vi "Compressor With Cylinder.vi"() -> ()   [LabVIEW 2013]
doc: "Compressor with Cylinder \n\nThis example shows how to control a compressor, extend and retract a cylinder, and optionally use a limit switch to retract automatically.\n\nThis example works with the NI 9403 module connected to a Digital Sidecar. The Digital Sidecar should have 12V applied to the WAGO connector. A SPIKE relay is used to turn the compressor on and off. The PWM type input on the SPIKE should be wired to RELAY 1 on the Digital Sidecar. The GND and 12V inputs on the SPIKE should get power from the battery through a 20A fuse on the Power Distribution Board. The M+ and M- outputs from the SPIKE should be wired to the compressor. Wire M+ to the red compressor wire, and M- to the black compressor wire. The Pressure Switch is wired to DIGITAL I/O 1. This input determines when the SPIKE relay gets energized to run the compressor. The Limit Switch is wired to DIGITAL I/O 2. It causes the cylinder to retract when the Auto Retract button is pressed.\n\nThis example also uses the Solenoid Breakout connected to the NI 9472 to control the SMC double solenoid valve. From the Solenoid Breakout, channel 1 is wired to terminal A on the valve, and channel 2 is wired to terminal B on the valve.\n\nRefer to the Pneumatics Manual for air connections. Your pneumatics setup should include a compressor, pressure switch, tank, regulator, valve, flow controls, cylinder, plug valve, etc.\n\nTo run this example you should have a pneumatic system with air pressure connected to the P input on the SMC double solenoid valve. The A output of the valve should be connected via a flow control to the backend of a cylinder. The B output of the valve should be connected via a flow control to the frontend of a cylinder. When the cylinder is extended, it should physically depress the Limit Switch.\n\nWith the VI running, pressing the Extend button will push the cylinder shaft out, and pressing the Retract button will pull it back. Notice that the Extend and Retract buttons have their Mechanical Action set to Latch When Pressed. This means they stay pressed (ON) until they are read by the program, then they return to the OFF position. This works because once the SMC solenoid valve is pulled one direction, it stays in that position until it is pulled in the opposite direction - it only needs to be momentarily energized. The Auto Retract button can be used to make the cylinder return automatically. With the Auto Retract button ON, pressing the Extend button will push the cylinder out, and it will retract when it hits the limit switch."
uses:
  <vilib>/Rock Robotics/WPI/Solenoid/WPI_SolenoidChannel.ctl
  <vilib>/Rock Robotics/SystemInterfaces/DIO/FPGA_DIOChannel.ctl
  <vilib>/Rock Robotics/SystemInterfaces/DIO/FPGA_DIORelayChannel.ctl
  <vilib>/Rock Robotics/SystemInterfaces/Typedef/FPGA_TypedefDigitalModule.ctl
  <vilib>/Rock Robotics/SystemInterfaces/Typedef/FPGA_TypedefSolenoidModule.ctl
  <vilib>/Rock Robotics/WPI/Solenoid/WPI_SolenoidValue.ctl
  <vilib>/Rock Robotics/WPI/Solenoid/WPI_SolenoidOpenDouble.vi
  <vilib>/Rock Robotics/WPI/Solenoid/WPI_SolenoidSetEnum.vi
panel:
  in  "Boolean":bool
  in  "Limit_Switch":T1=enum."DIO 10"
  in  "2nd_position":bool
  in  "Shooter":bool
  in  "Load":bool
  in  "Small_Cylinder_Extend":T2=enum."Solenoid 4"
  in  "Small_Cylinder_Retract":T2=enum."Solenoid 3"
  out "Compressor Running?":bool
  in  "Solenoid Module":T3
  in  "Large_Cylinder_Extend":T2=enum."Solenoid 2"
  in  "Switch and Relay Module":T4
  in  "RelayChannel":T5=enum."Relay 2"
  in  "Pressure Switch Channel":T1=enum."DIO 5"
  in  "Large_Cylinder_Retract":T2
  out "Compressor Enabled?":bool
  in  "stop":bool
  # "Set these inputs before running."
  # "These can be set while running."
  # "Output information."
  # "Wiring Diagram for Digital Sidecar connected to an NI 9403"
  # "when extended, the cylinder should depress this"
  # "Limit\nSwitch"
  # "(-)"
  # "B"
  # "A"
  # "8\n7\n6\n5\n4\n3\n2\n1"
  # "RELAY"
  # "Pressure\nSwitch"
  # "Connect\nPower\nHere"
  # "GND"
  # "M-"
  # "Connect\nCompressor\nHere"
  # "SPIKE"
  # "12V"
  # "M+"
  # "B"
  # "20A"
  # "fuse"
  # "SPIKE Relay"
  # "PWM cable"
  # "COM"
  # "NC"
  # "NO"
  # "NC"
  # "C"
  # "PWR"
  # "SIG"
  # "(-)"
  # "14\n13\n12\n11\n10\n9\n8\n7\n6\n5\n4\n3\n2\n1"
  # "DIGITAL I/O"
  # "Digital Sidecar"
  # "Wiring Diagram for Solenoid Breakout connected to an NI 9472"
  # "GND"
  # "SIG"
  # "8\n7\n6\n5\n4\n3\n2\n1"
  # "+"
  # "12V from\nbattery"
  # "-"
  # "tubing port for retract side of cylinder"
  # "tubing port for extend side of cylinder"
  # "\"power good\"\n  LED"
  # "SMC double solenoid valve"
  # "B"
  # "A"
  # "B"
  # "A"
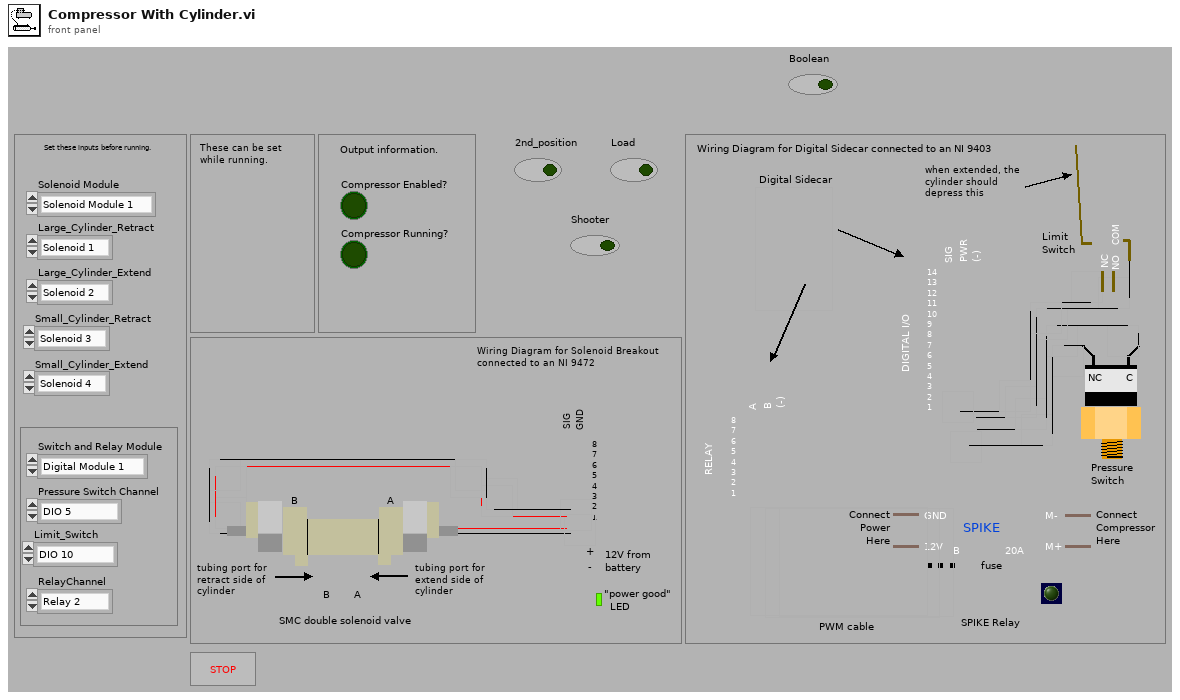
[diagram p1: front panel]
types:
  T1 = typedef "FPGA_DIOChannel.ctl" = enum8{"DIO 1", "DIO 2", "DIO 3", "DIO 4", "DIO 5", "DIO 6", "DIO 7", "DIO 8", "DIO 9", "DIO 10", "DIO 11", "DIO 12", "DIO 13", "DIO 14", "Invalid"}
  T2 = typedef "WPI_SolenoidChannel.ctl" = enum8{"Solenoid 1", "Solenoid 2", "Solenoid 3", "Solenoid 4", "Solenoid 5", "Solenoid 6", "Solenoid 7", "Solenoid 8", "Invalid"}
  T3 = typedef "FPGA_TypedefSolenoidModule.ctl" = enum16{"Solenoid Module 1", "Solenoid Module 2"}
  T4 = typedef "FPGA_TypedefDigitalModule.ctl" = enum16{"Digital Module 1", "Digital Module 2"}
  T5 = typedef "FPGA_DIORelayChannel.ctl" = enum8{"Relay 1", "Relay 2", "Relay 3", "Relay 4", "Relay 5", "Relay 6", "Relay 7", "Relay 8", "Invalid"}
  T6 = typedef "WPI_CompressorDevRef.ctl" = cluster{"DevStatus":errorcluster, "DigitalInputDevRef":T7, "RelayDevRef":T8}
  T7 = typedef "WPI_DigitalInputDevRef.ctl" = cluster{"DevStatus":errorcluster, "DIO Channel":T1, "Digital Module":T4}
  T8 = typedef "WPI_RelayDevRef.ctl" = cluster{"DevStatus":errorcluster, "Relay Channel":T5, "Digital Module":T4, "Relay Direction":T9}
  T9 = typedef "WPI_RelayDirection.ctl" = enum16{"Both directions", "Forward only", "Reverse only"}
  T10 = typedef "WPI_SolenoidDevRef.ctl" = cluster{"DevStatus":errorcluster, "Solenoid Module":T3, "Forward Solenoid Channel":T2, "Reverse Solenoid Channel":T2}
  T11 = typedef "WPI_SolenoidValue.ctl" = enum16{"Off", "On", "Forward", "Reverse"}
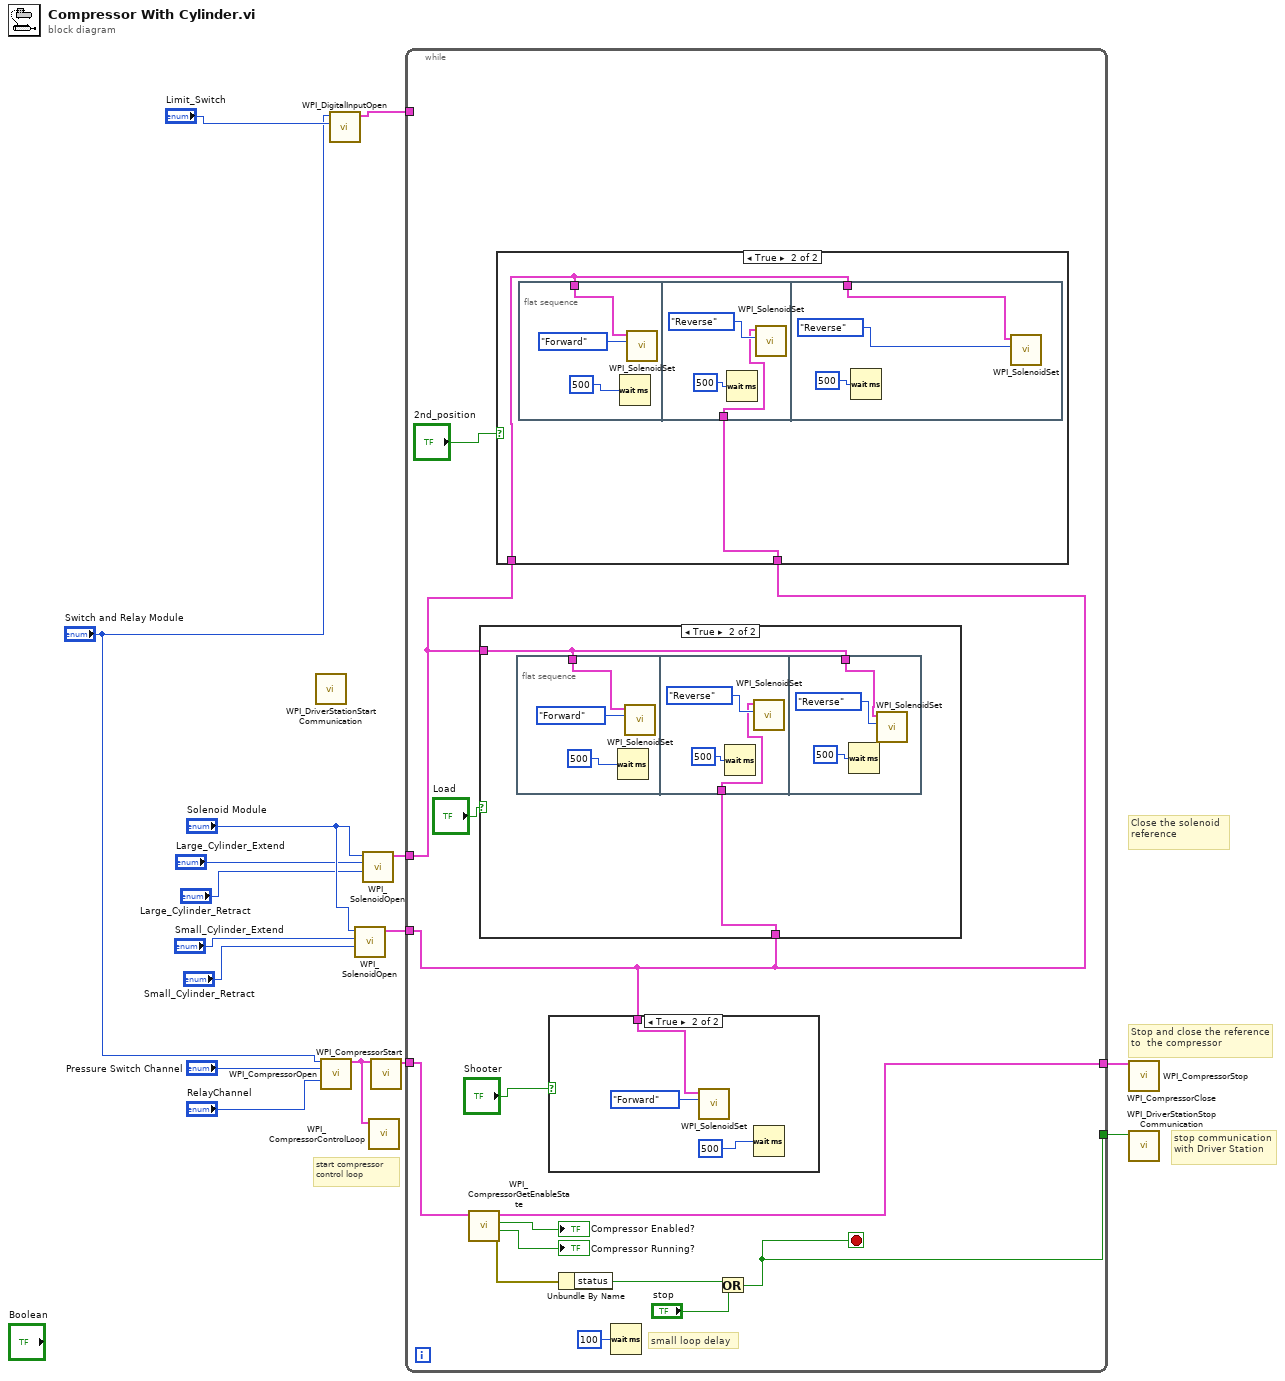
[diagram p0: block diagram]
diagram:
  # "start compressor control loop"
  # "Close the solenoid\nreference"
  # "stop communication with Driver Station"
  # "Stop and close the reference to  the compressor"
  n1 = call <vilib>:"WPI_DriverStationStart Communication.vi"() -> ()  [unwired: 1 in, 11 out]
  n2 = call <vilib>:"WPI_CompressorOpen.vi"("Pressure Switch Digital Module (Module 1)"="Switch and Relay Module", "Pressure Switch DIO Channel"="Pressure Switch Channel", "Relay Channel"="RelayChannel") -> ("CompressorDevRef"=w10:T6)  [unwired: 2 in, 10 out]
  n3 = call <vilib>:"WPI_DigitalInputOpen.vi"("DIO Channel"="Limit_Switch", "Digital Module (Module 1)"="Switch and Relay Module") -> ("DigitalInputDevRef"=w3:T7)  [unwired: 8 in, 1 out]
  n4 = call-poly <vilib>:"WPI_SolenoidOpen.vi"("Reverse Solenoid Channel"="Small_Cylinder_Retract", "Forward Solenoid Channel"="Small_Cylinder_Extend", "Solenoid Module (Module 1)"="Solenoid Module") -> ("SolenoidDevRef"=w8:T10)  [unwired: 1 in, 7 out]
  n5 = call-poly <vilib>:"WPI_SolenoidOpen.vi"("Reverse Solenoid Channel"="Large_Cylinder_Retract", "Forward Solenoid Channel"="Large_Cylinder_Extend", "Solenoid Module (Module 1)"="Solenoid Module") -> ("SolenoidDevRef"=w11:T10)  [unwired: 1 in, 7 out]
  n6 = call <vilib>:"WPI_CompressorControlLoop.vi"("CompressorDevRef"=w10) -> ()  [unwired: 11 in]
  n7 = call <vilib>:"WPI_CompressorStart.vi"("CompressorDevRef"=w10) -> ("CompressorDevRef"=w16:T6)  [unwired: 1 in, 9 out]
  n8 = while {
    tunnel: w16 -> [w31]
    tunnel: [w30] -> w15
    tunnel: [w28] -> w12
    tunnel: w11 -> [w19]
    tunnel: w8 -> [w18]
    tunnel: w3 -> [_]
    stop <- w28 stop-if-true
    # "small loop delay"
    n9 = call <vilib>:"WPI_CompressorGetEnableState.vi"("CompressorDevRef"=w31) -> ("error out"=w26:errorcluster, "Compressor Running"=→"Compressor Running?":bool, "Enabled"=→"Compressor Enabled?":bool, "CompressorDevRef"=w30:T6)  [unwired: 1 in, 6 out]
    n10 = case shown="True" "Load" {
      tunnel: w19 -> [_ w47]
      tunnel: w18 -> [_ w46]
      frame False {
      }
      frame True {
        n11 = flat-sequence {
          tunnel: w47 -> [w48]
          tunnel: w46 -> [w51]
          tunnel: w47 -> [w54]
          frame #0 {
            n12 = Wait (ms)(milliseconds to wait=500) -> ()  [unwired: 1 out]
            n13 = call-poly <vilib>:"WPI_SolenoidSet.vi"("Value"=WPI_SolenoidValue."Forward", "SolenoidDevRef"=w48) -> ()  [unwired: 1 in, 9 out]
          }
          frame #1 {
            n14 = Wait (ms)(milliseconds to wait=500) -> ()  [unwired: 1 out]
            n15 = call-poly <vilib>:"WPI_SolenoidSet.vi"("Value"=WPI_SolenoidValue."Reverse", "SolenoidDevRef"=w51) -> ()  [unwired: 1 in, 9 out]
          }
          frame #2 {
            n16 = Wait (ms)(milliseconds to wait=500) -> ()  [unwired: 1 out]
            n17 = call-poly <vilib>:"WPI_SolenoidSet.vi"("Value"=WPI_SolenoidValue."Reverse", "SolenoidDevRef"=w54) -> ()  [unwired: 1 in, 9 out]
          }
        }
      }
    }
    n18 = case shown="True" "2nd_position" {
      tunnel: w18 -> [_ w33]
      tunnel: w19 -> [_ w32]
      frame False {
      }
      frame True {
        n19 = flat-sequence {
          tunnel: w32 -> [w34]
          tunnel: w33 -> [w37]
          tunnel: w32 -> [w41]
          frame #0 {
            n20 = Wait (ms)(milliseconds to wait=500) -> ()  [unwired: 1 out]
            n21 = call-poly <vilib>:"WPI_SolenoidSet.vi"("Value"=WPI_SolenoidValue."Forward", "SolenoidDevRef"=w34) -> ()  [unwired: 1 in, 9 out]
          }
          frame #1 {
            n22 = Wait (ms)(milliseconds to wait=500) -> ()  [unwired: 1 out]
            n23 = call-poly <vilib>:"WPI_SolenoidSet.vi"("Value"=WPI_SolenoidValue."Reverse", "SolenoidDevRef"=w37) -> ()  [unwired: 1 in, 9 out]
          }
          frame #2 {
            n24 = Wait (ms)(milliseconds to wait=500) -> ()  [unwired: 1 out]
            n25 = call-poly <vilib>:"WPI_SolenoidSet.vi"("Value"=WPI_SolenoidValue."Reverse", "SolenoidDevRef"=w41) -> ()  [unwired: 1 in, 9 out]
          }
        }
      }
    }
    n26 = case shown="True" "Shooter" {
      tunnel: w18 -> [_ w44]
      frame False {
      }
      frame True {
        n27 = call-poly <vilib>:"WPI_SolenoidSet.vi"("Value"=WPI_SolenoidValue."Forward", "SolenoidDevRef"=w44) -> ()  [unwired: 1 in, 9 out]
        n28 = Wait (ms)(milliseconds to wait=500) -> ()  [unwired: 1 out]
      }
    }
    n29 = Unbundle By Name(w26) -> ("status"=w25:bool)
    n30 = Wait (ms)(milliseconds to wait=u32 100) -> ()  [unwired: 1 out]
    n31 = Or(x=w25, y="stop") -> (x .or. y?=w28:bool)
  }
  n32 = call <vilib>:"WPI_CompressorStop.vi"("CompressorDevRef"=w15) -> ("CompressorDevRef"=w17:T6)  [unwired: 1 in, 9 out]
  n33 = call <vilib>:"WPI_CompressorClose.vi"("CompressorDevRef"=w17) -> ()  [unwired: 1 in, 10 out]
  n34 = call <vilib>:"WPI_DriverStationStop Communication.vi"("StopCommunication"=w12) -> ()  [unwired: 1 in, 10 out]
